vi "GUI Configuration Loop.vi"(7 "FOFB Controller IP":string, 8 "error in (no error)":errorcluster, 9 "FOFB GUI":T1, 10 "TCP Listening Timeout":i32, 11 "Configuration GUI TCP Port":u16) -> (0 "error out":errorcluster)   [LabVIEW 2011, in "User Interface VIs.lvlib"]
uses:
  User Interface VIs.lvlib
  Types Definitions/Type FOFB GUI.ctl
  Types Definitions/Type FOFB Parameters.ctl
  Types Definitions/Type Network Configuration.ctl
  Types Definitions/Type FA Configuration.ctl
  Types Definitions/Type Response Matrix Measurement Configuration.ctl
  Types Definitions/Type Correction Algorithm Configuration.ctl
  Types Definitions/Type Acquisition Network Configuration.ctl
  Types Definitions/Type Actuation Network Configuration.ctl
  Types Definitions/Type Configuration Loop Mode.ctl
  Types Definitions/Type Configuration Data (GUI to Controller).ctl
  Types Definitions/Type Monitoring Data.ctl
  Types Definitions/Type Diagnostics Data.ctl
  Types Definitions/Type CPU Loads Array.ctl
  Types Definitions/Type CPU Loads.ctl
  Types Definitions/Type Diagnostics Sample.ctl
  Types Definitions/Type Monitoring Sample.ctl
  <vilib>/Platform/TimedLoop/XDataNode/timing_clust.ctl
  <vilib>/Platform/TimedLoop/XDataNode/nitl_modes.ctl
  <vilib>/Platform/TimedLoop/XDataNode/wakeup.ctl
  Types Definitions/Type Configuration Change Acknowledge (Controller to GUI).ctl
  <vilib>/Platform/TimedLoop/XDataNode/XDataNode.xnode
  Type Definitions.lvlib
  Misc VIs.lvlib
  <vilib>/Platform/TimedLoop/XDataNode/XDNodeRunTimeDep.lvlib
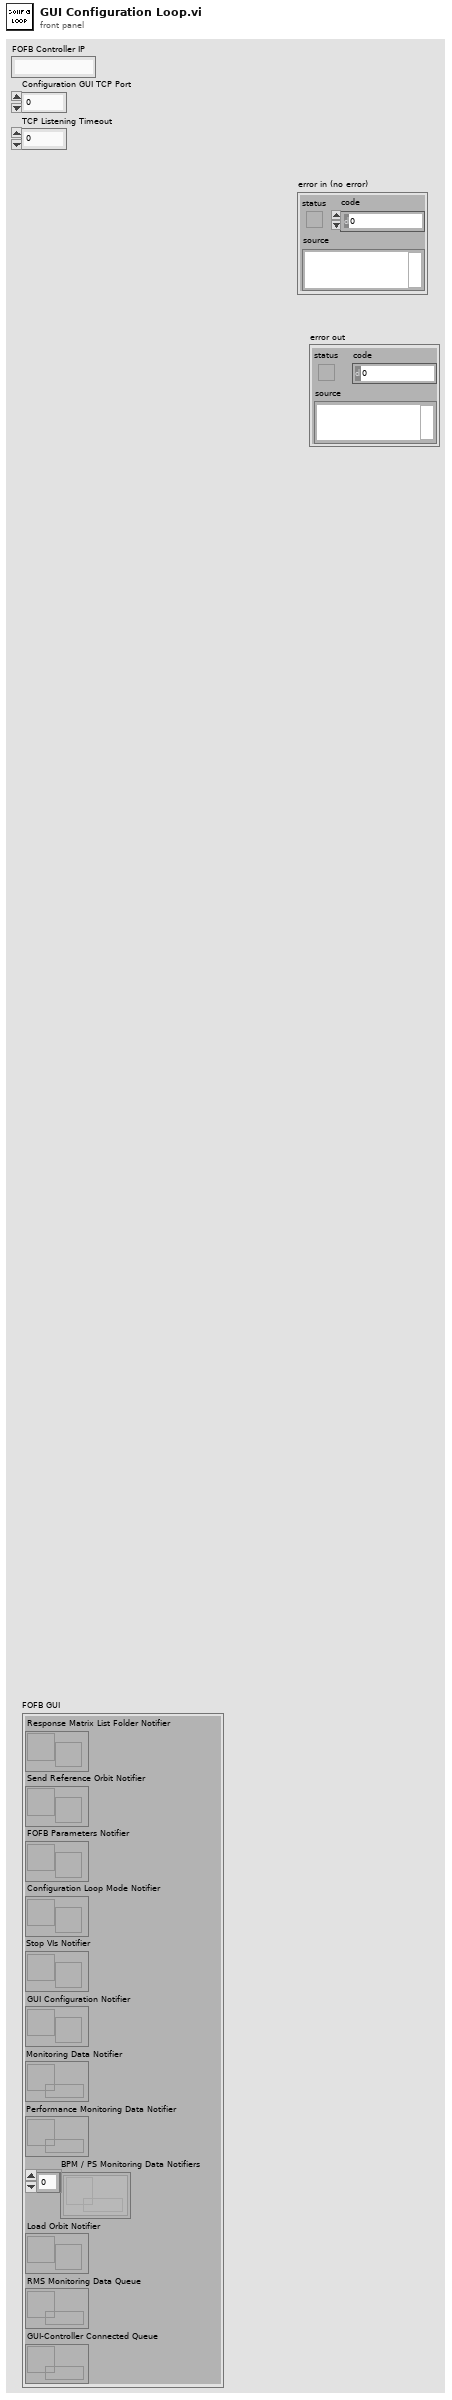
[diagram p1: front panel]
types:
  T1 = typedef "Type Definitions.lvlib/Type FOFB GUI.ctl" = cluster{"Response Matrix List Folder Notifier":refnum<notifier>, "Send Reference Orbit Notifier":refnum<notifier>, "FOFB Parameters Notifier":refnum<notifier>, "Configuration Loop Mode Notifier":refnum<notifier>, "Stop VIs Notifier":refnum<notifier>, "GUI Configuration Notifier":refnum<notifier>, "Monitoring Data Notifier":refnum<queue>, "Performance Monitoring Data Notifier":refnum<queue>, "BPM / PS Monitoring Data Notifiers":refnum<queue>[], "Load Orbit Notifier":refnum<notifier>, "RMS Monitoring Data Queue":refnum<queue>, "GUI-Controller Connected Queue":refnum<queue>}
  T2 = enum16{"Idle", "Wait Connection", "Read Data", "Process Data", "Write Data", "Close Connection"}
  T3 = typedef "XDNodeRunTimeDep.lvlib/timing_clust.ctl" = cluster{"Expected End [f-1]":u64, "Actual End [f-1]":u64, "Finished Late? [f-1]":bool, "Expected End [i-1]":u64, "Actual End [i-1]":u64, "Finished Late? [i-1]":bool, "Expected Start [i]":u64, "Actual Start [i]":u64, "Expected Start [f]":u64, "Actual Start [f]":u64, "Source Name":string, "Structure Name":string, "Period":i64, "Deadline":i64, "Offset":i64, "Start":i64, "Priority":i32, "Timeout":i32, "Mode":T4, "Wakeup Reason":T5, "Error":errorcluster, "Source Type":string, "Secondary Source Type":string, "Global End Time":u64, "Global Start Time":u64, "Frame Duration":u64, "Iteration Duration":u64, "Assigned CPU":i32, "I/O Scan Engine Mode":u32}
  T4 = typedef "XDNodeRunTimeDep.lvlib/nitl_modes.ctl" = enum32{"No Change", "Process missed periods, maintain original phase", "Discard missed periods, maintain original phase", "Process missed periods, ignore original phase", "Discard missed periods, ignore original phase"}
  T5 = typedef "XDNodeRunTimeDep.lvlib/wakeup.ctl" = enum32{"Normal", "Aborted", "Asynchronous wakeup", "Timing source error", "Timed loop error", "Timeout"}
  T6 = typedef "Type Definitions.lvlib/Type Configuration Data (GUI to Controller).ctl" = cluster{"Update Controller Soft Configuration":bool[], "Trigger RT Execution Trace":string[], "Reference Orbit":dbl[], "Request Response Matrix Folder List":bool[], "Request FOFB Parameters":bool[], "FOFB Parameters":T7[]}
  T7 = typedef "Type Definitions.lvlib/Type FOFB Parameters.ctl" = cluster{"Network":T8, "Fast Acquisition":T9, "Response Matrix Measurement":T10, "Correction Algorithm":T11, "Acquisition Network":T12, "Actuation Network":T13}
  T8 = typedef "Type Definitions.lvlib/Type Network Configuration.ctl" = cluster{"FOFB Controller IP":string, "LNLS Control Network IP":string, "LNLS Control Network Power Supplies TCP Port":u16, "LNLS Control Network FOFB Configuration TCP Port":u16, "Data Server TCP Port":u16, "Monitoring Data TCP Port":u16, "Configuration GUI TCP Port":u16, "TCP Listening Timeout":i32}
  T9 = typedef "Type Definitions.lvlib/Type FA Configuration.ctl" = cluster{"Acquisition Period":u32, "Data Buffer Size":u32, "Monitoring Period":u32}
  T10 = typedef "Type Definitions.lvlib/Type Response Matrix Measurement Configuration.ctl" = cluster{"Step Amplitude":dbl, "Time Between Steps":u32, "Step Duration":u32, "Number of Averages":u32}
  T11 = typedef "Type Definitions.lvlib/Type Correction Algorithm Configuration.ctl" = cluster{"Correction Period":u32, "Reference Orbit Path":path, "Response Matrix Path":path, "Correction Matrix Path":path, "Horizontal Correction Factor":dbl, "Vertical Correction Factor":dbl, "Beam Current FOFB Threshold":dbl, "Decouple H-V":bool, "Use Additional BPM LPF":bool, "BPM LPF Cutoff":dbl}
  T12 = typedef "Type Definitions.lvlib/Type Acquisition Network Configuration.ctl" = cluster{"Chassis Name":string, "Variables":cluster{"Variable Name":string, "Matrix Order":u32, "Location":dbl, "Plane":enum8{"H", "V"}, "On Correction":bool}[]}[]
  T13 = typedef "Type Definitions.lvlib/Type Actuation Network Configuration.ctl" = cluster{"Chassis Name":string, "Variables":cluster{"Variable Name":string, "Matrix Order":u32, "RMM Step Factor":dbl, "Plane":enum8{"H", "V"}, "On Correction":bool, "Kc":dbl, "Ti":dbl, "Td":dbl}[]}[]
  T14 = typedef "Type Definitions.lvlib/Type Configuration Change Acknowledge (Controller to GUI).ctl" = cluster{"Request Response Matrix List Folder":string[], "FOFB Parameters":T7[]}
  T15 = typedef "Type Definitions.lvlib/Type Configuration Loop Mode.ctl" = enum8{"Operation Mode", "Request FOFB Parameters", "Send New FOFB Parameters", "Send Reference Orbit", "Request Response Matrix List Folder"}
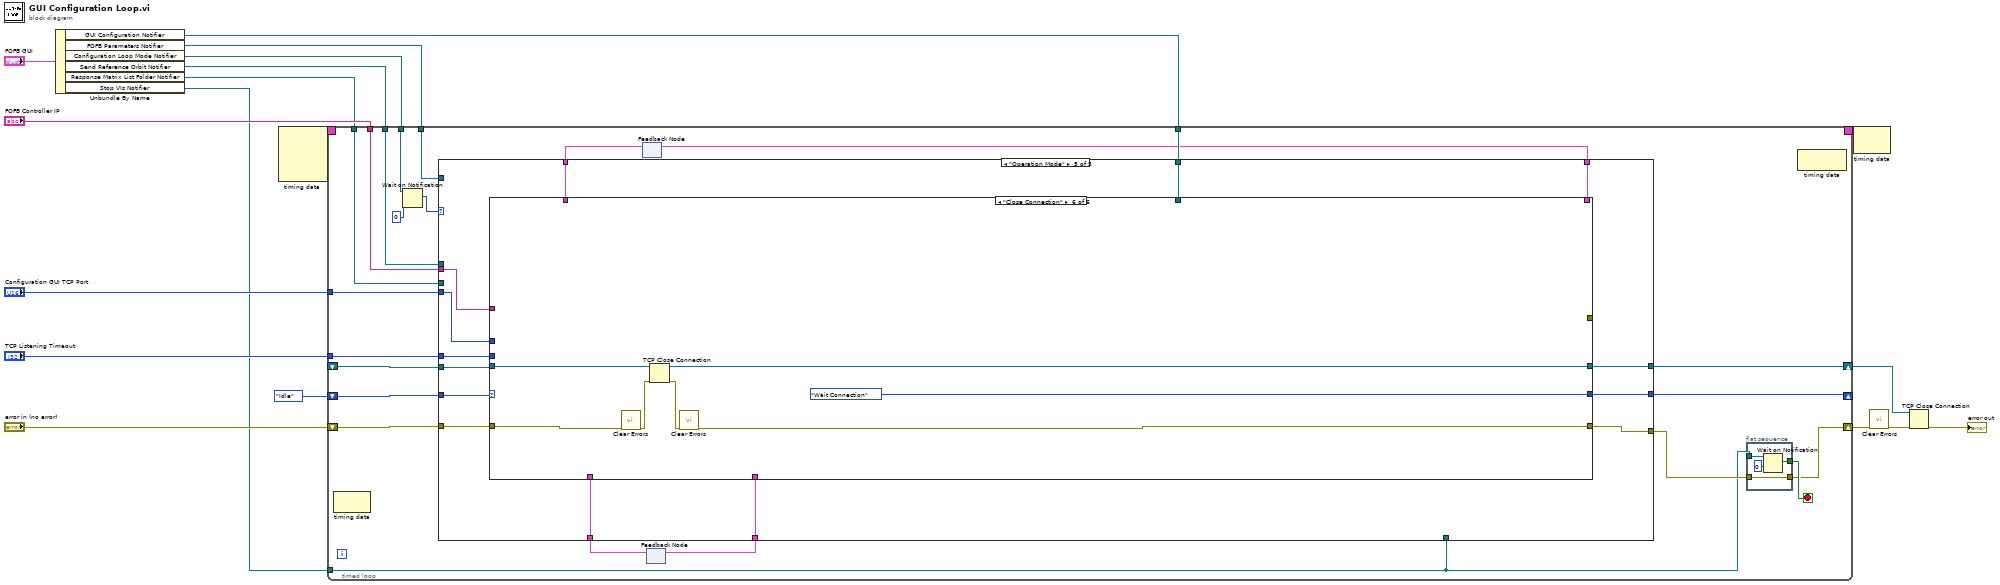
[diagram p0: block diagram]
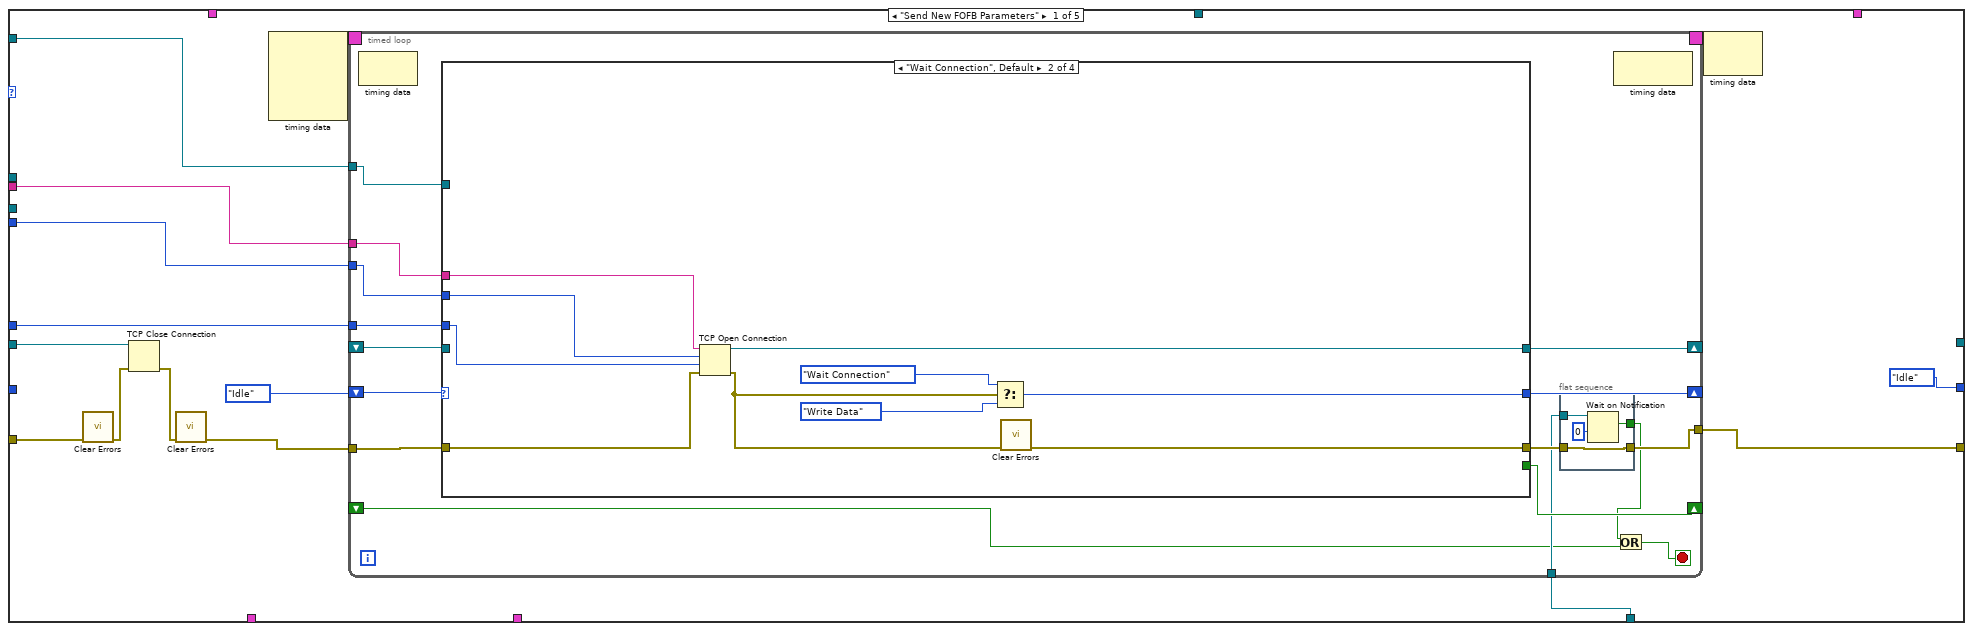
[diagram p2: hidden frame]
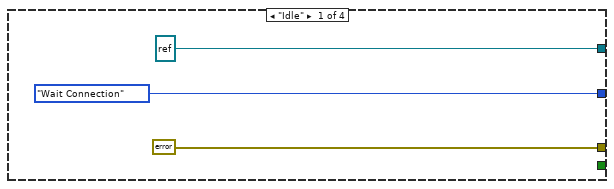
[diagram p3: hidden frame]
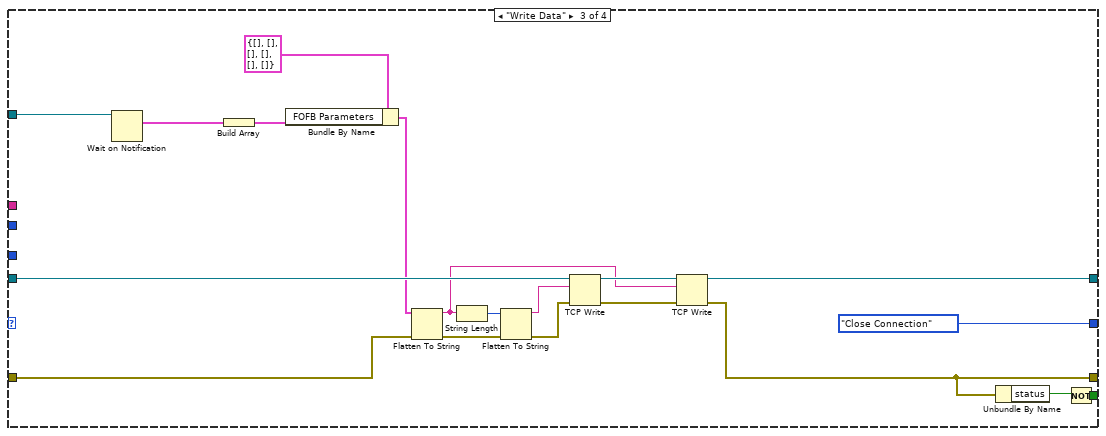
[diagram p4: hidden frame]
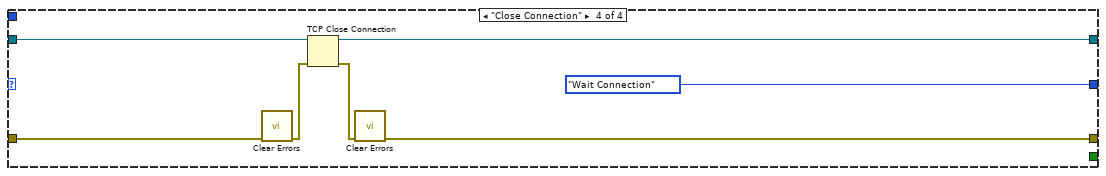
[diagram p5: hidden frame]
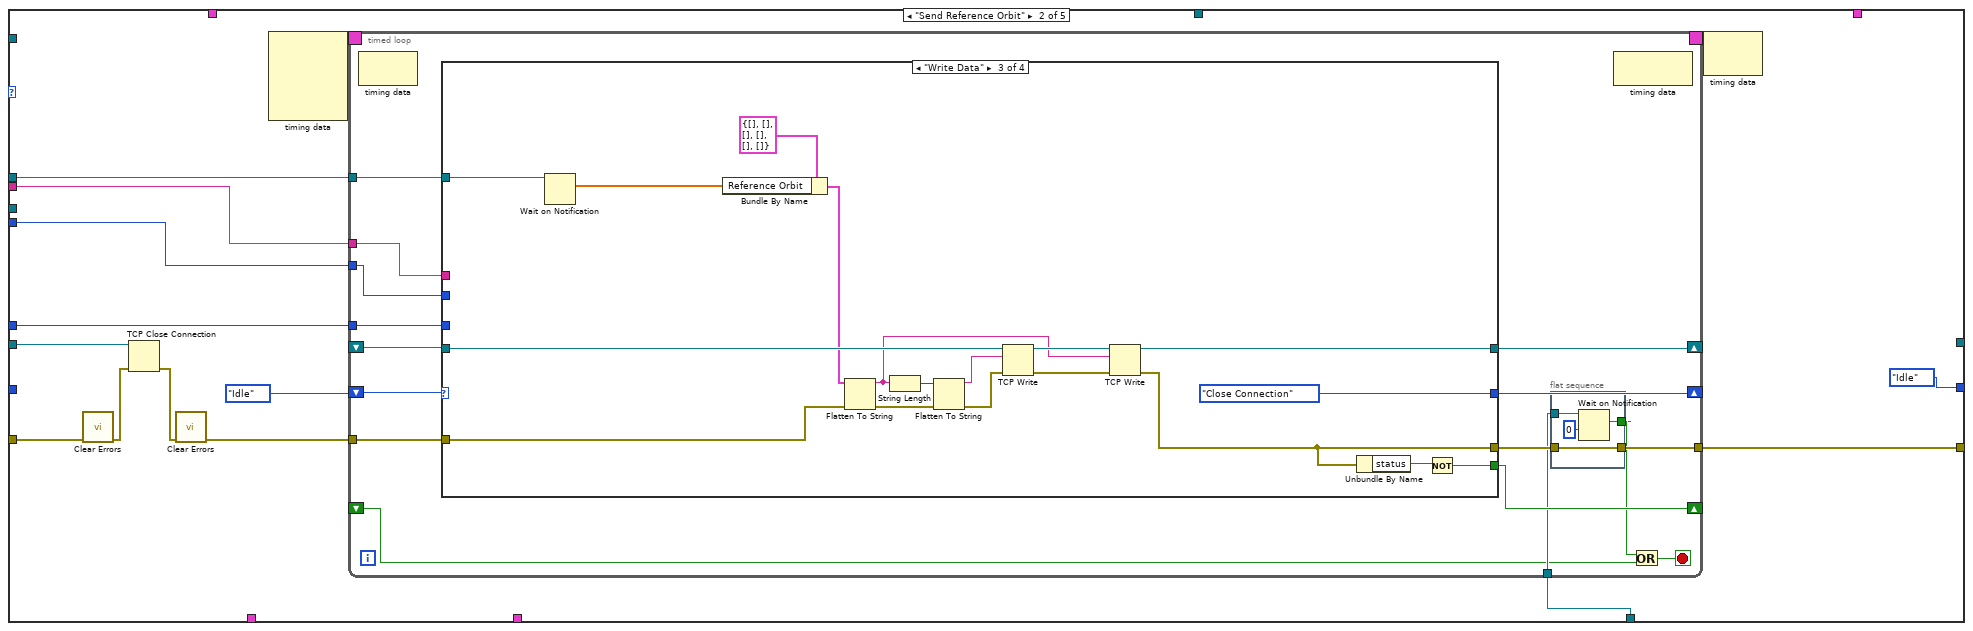
[diagram p6: hidden frame]
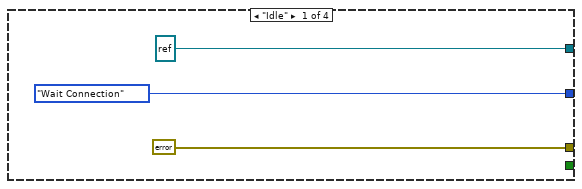
[diagram p7: hidden frame]
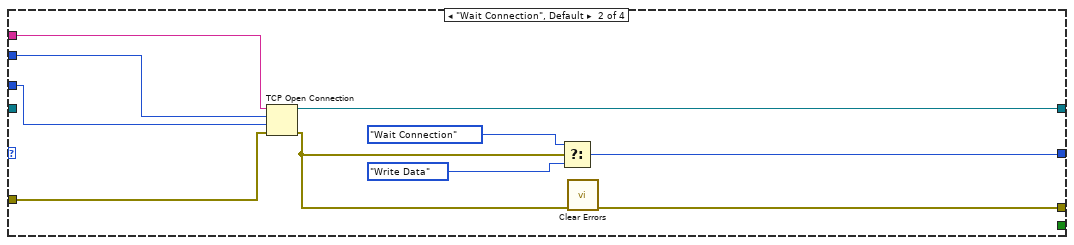
[diagram p8: hidden frame]
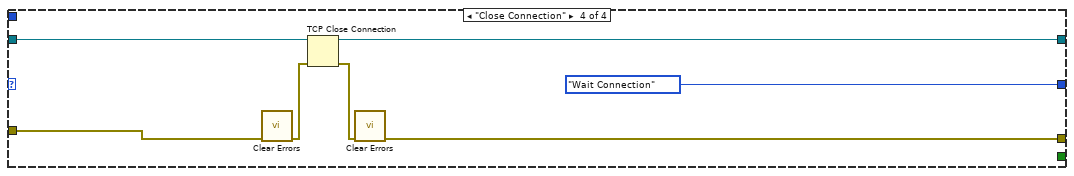
[diagram p9: hidden frame]
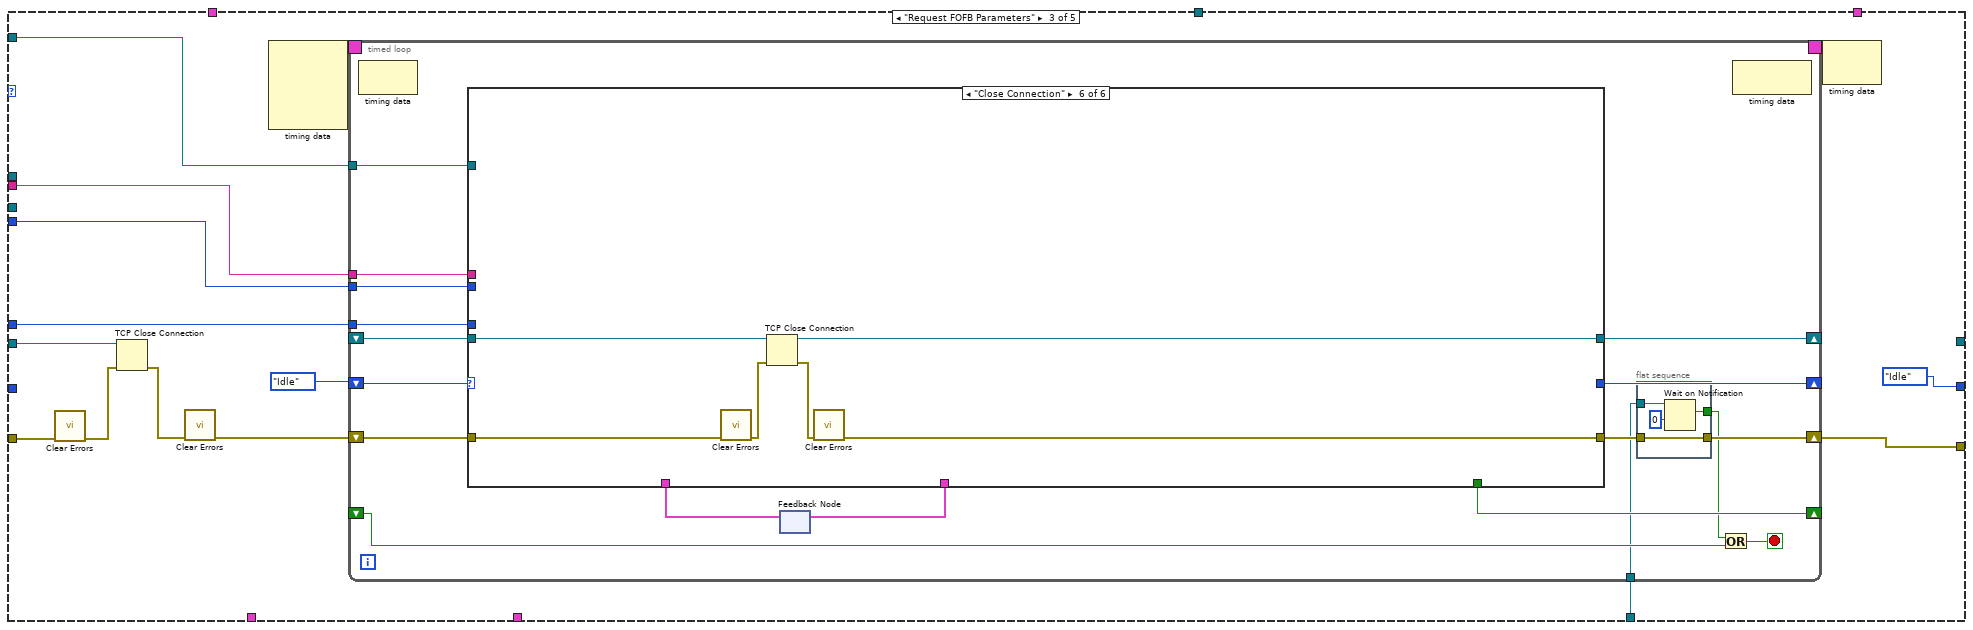
[diagram p10: hidden frame]
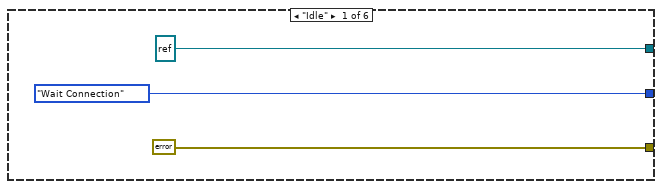
[diagram p11: hidden frame]
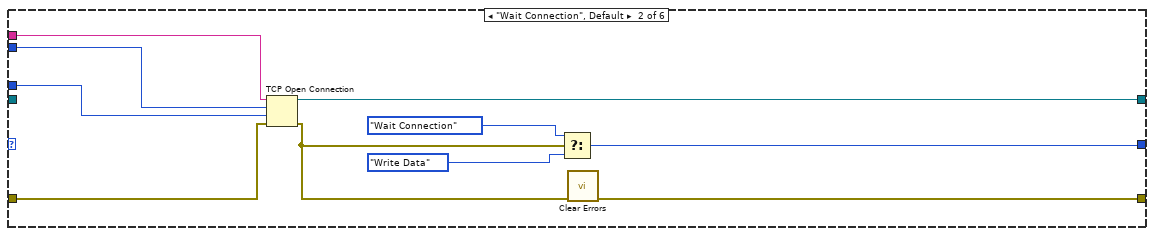
[diagram p12: hidden frame]
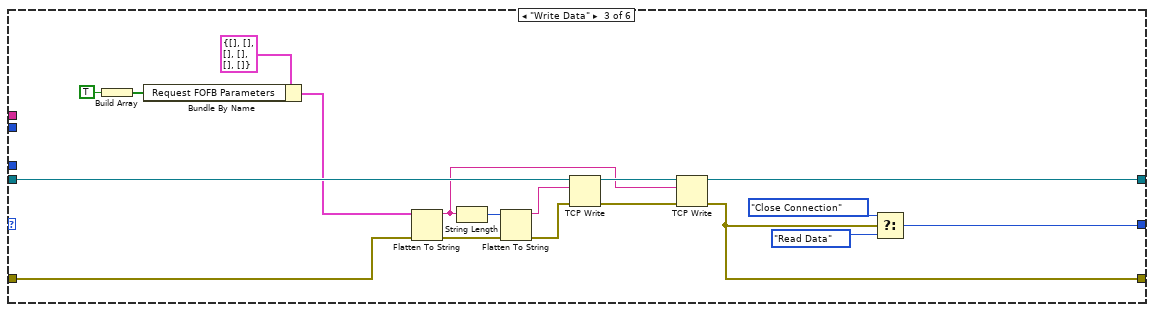
[diagram p13: hidden frame]
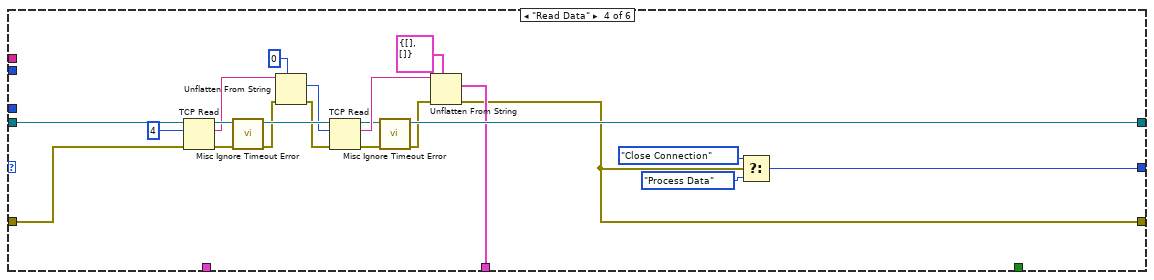
[diagram p14: hidden frame]
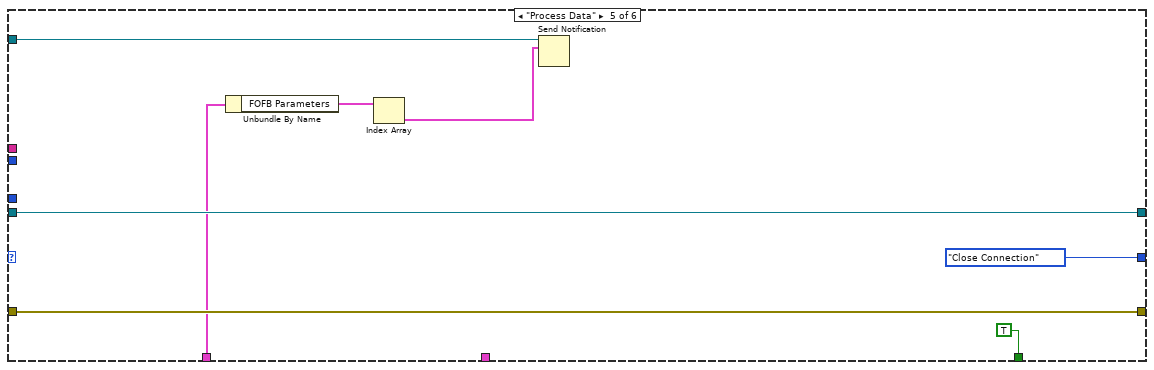
[diagram p15: hidden frame]
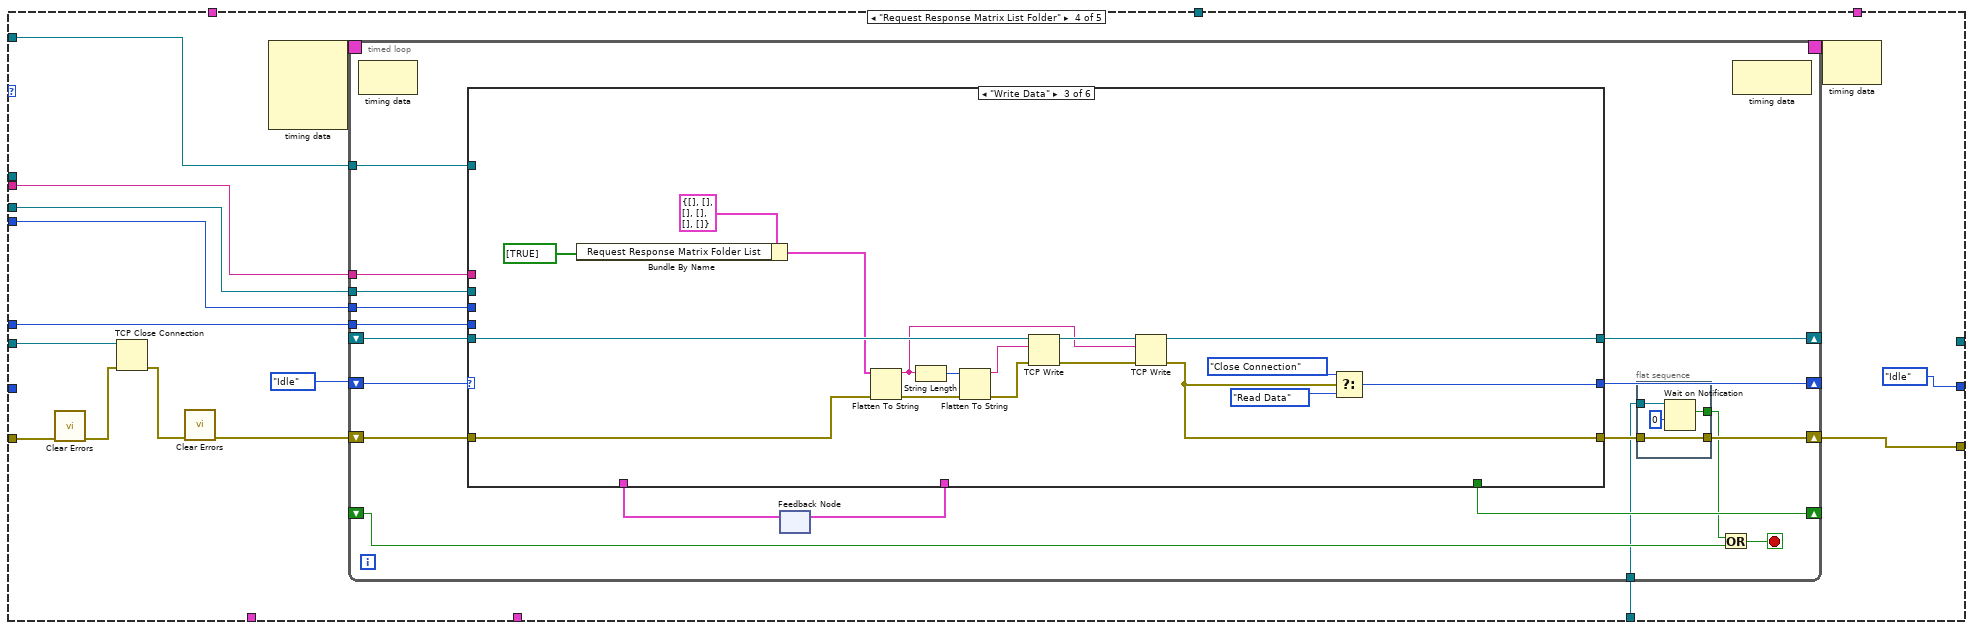
[diagram p16: hidden frame]
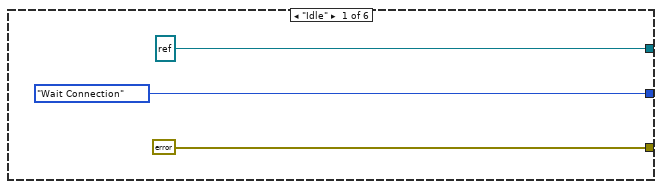
[diagram p17: hidden frame]
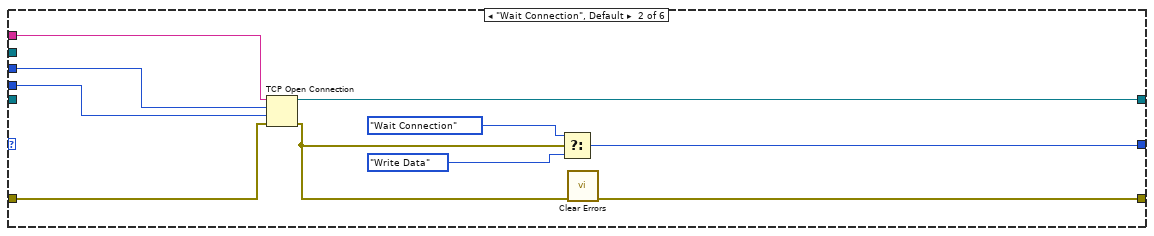
[diagram p18: hidden frame]
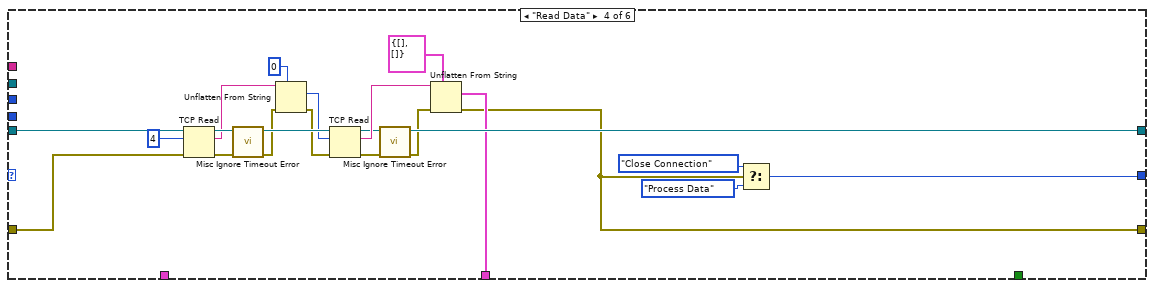
[diagram p19: hidden frame]
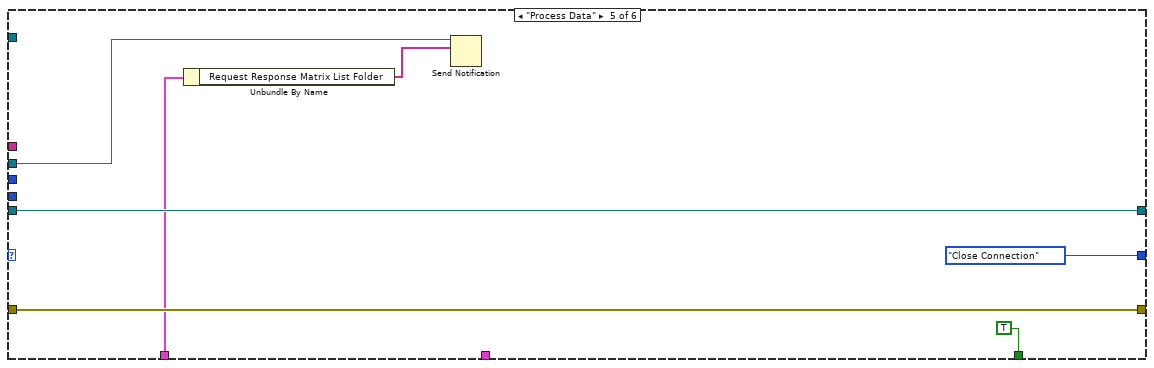
[diagram p20: hidden frame]
diagram:
  n1 = Unbundle By Name("FOFB GUI") -> ("GUI Configuration Notifier"=w9:refnum<notifier>, "FOFB Parameters Notifier"=w4:refnum<notifier>, "Configuration Loop Mode Notifier"=w12:refnum<notifier>, "Send Reference Orbit Notifier"=w3:refnum<notifier>, "Response Matrix List Folder Notifier"=w1:refnum<notifier>, "Stop VIs Notifier"=w2:refnum<notifier>)
  n2 = node-c288() -> (w16:T3)  [unwired: 4 in]
  n3 = timed-loop {
    timing: w16 -> [_]
    timing-out: [_] -> w15
    tunnel: w4 -> [w19]
    tunnel: "FOFB Controller IP" -> [w39]
    tunnel: "Configuration GUI TCP Port" -> [w38]
    tunnel: "TCP Listening Timeout" -> [w37]
    tunnel: w12 -> [w20]
    shift-right: [w33] -> w6
    shift-left: "error in (no error)" -> [w35]
    tunnel: w2 -> [w23]
    tunnel: w9 -> [w32]
    shift-right: [w30] -> _
    shift-left: T2."Idle" ("f") -> [w31]
    shift-right: [w28] -> w5
    shift-left: _ -> [w29]
    tunnel: w3 -> [w22]
    tunnel: w1 -> [w21]
    stop <- w36 stop-if-true
    n4 = node-c288() -> ()  [unwired: 1 in, 1 out]
    n5 = Wait on Notification(notifier=w20, timeout in ms (-1)=0) -> (notification=w41:T15)  [unwired: 2 in, 3 out]
    n6 = feedback #1() -> (w25:T6)  [unwired: 1 in]
    n7 = feedback #2() -> (w27:T14)  [unwired: 1 in]
    n8 = case shown="\"Operation Mode\"" w41 {
      tunnel: w35 -> [w49 w128 w203 w310 w417]
      tunnel: w19 -> [w60 _ w215 w322 _]
      tunnel: w39 -> [w56 w135 w211 w318 w420]
      tunnel: w38 -> [w55 w134 w210 w317 w419]
      tunnel: w37 -> [w54 w133 w209 w316 w418]
      tunnel: [w53 w132 w208 w315 w426] -> w34
      tunnel: w32 -> [_ _ _ _ w425]
      tunnel: w31 -> [_ _ _ _ w424]
      tunnel: [T2."Idle" ("f") T2."Idle" ("f") T2."Idle" ("f") T2."Idle" ("f") w423] -> w30
      tunnel: w29 -> [w47 w126 w204 w311 w422]
      tunnel: [_ _ _ _ w421] -> w28
      tunnel: w27 -> [_ _ _ _ w416]
      tunnel: [_ _ _ _ w415] -> w26
      tunnel: w25 -> [_ _ _ _ w414]
      tunnel: [_ _ _ _ w413] -> w24
      tunnel: w23 -> [w46 w124 w201 w308 _]
      tunnel: w22 -> [_ w125 _ _ _]
      tunnel: w21 -> [_ _ _ w307 _]
      frame "Send New FOFB Parameters" {
        n9 = call <vilib>:"Clear Errors.vi"("error in (no error)"=w49) -> ("error out"=w50:errorcluster)  [unwired: 6 in]
        n10 = TCP Close Connection(connection ID=w47, error in (no error)=w50) -> (error out=w51:errorcluster)  [unwired: 1 in, 1 out]
        n11 = call <vilib>:"Clear Errors.vi"("error in (no error)"=w51) -> ("error out"=w48:errorcluster)  [unwired: 6 in]
        n12 = node-c288() -> (w59:T3)  [unwired: 4 in]
        n13 = timed-loop {
          timing: w59 -> [_]
          timing-out: [_] -> w58
          tunnel: w48 -> [w76]
          tunnel: [w65] -> w53
          tunnel: w60 -> [w75]
          shift-right: [w71] -> _
          shift-left: T2."Idle" ("f") -> [w74]
          shift-right: [w72] -> _
          shift-left: _ -> [w73]
          tunnel: w56 -> [w70]
          tunnel: w55 -> [w69]
          tunnel: w54 -> [w68]
          shift-right: [w67] -> _
          shift-left: _ -> [w62]
          tunnel: w46 -> [w64]
          stop <- w61 stop-if-true
          n14 = node-c288() -> ()  [unwired: 1 in, 1 out]
          n15 = case shown="\"Wait Connection\", Default" w74 {
            tunnel: [refnum<k5> refnum ("connection ID") w89 w112 w119] -> w72
            tunnel: [T2."Wait Connection" ("f") w93 T2."Close Connection" ("f") T2."Wait Connection" ("f")] -> w71
            tunnel: [errorcluster {"status"=FALSE, "code"=0, "source"=""} ("error out") w92 w99 w118] -> w66
            tunnel: w76 -> [_ w87 w110 w113]
            tunnel: w73 -> [_ _ w111 w114]
            tunnel: w75 -> [_ _ w98 _]
            tunnel: w70 -> [_ w86 _ _]
            tunnel: w69 -> [_ w85 _ _]
            tunnel: w68 -> [_ w84 _ _]
            tunnel: [_ _ w100 _] -> w67
            frame "Idle" {
            }
            frame "Wait Connection", Default {
              n16 = TCP Open Connection(address=w86, remote port or service name=w85, timeout ms (60000)=w84, error in (no error)=w87) -> (connection ID=w89:refnum<k5>, error out=w88:errorcluster)  [unwired: 1 in]
              n17 = Select(t=T2."Wait Connection" ("f"), s=w88, f=T2."Write Data") -> (s? t:f=w93:T2)
              n18 = call <vilib>:"Clear Errors.vi"("error in (no error)"=w88) -> ("error out"=w92:errorcluster)  [unwired: 6 out]
            }
            frame "Write Data" {
              n19 = Wait on Notification(notifier=w98) -> (notification=w102:T7)  [unwired: 3 in, 3 out]
              n20 = Build Array(w102) -> (w94:T7[])
              n21 = Bundle By Name(cluster=T6 {"Update Controller Soft Configuration"=[], "Trigger RT Execution Trace"=[], "Reference Orbit"=[], "Request Response Matrix Folder List"=[], "Request FOFB Parameters"=[], "FOFB Parameters"=[]} ("Configuration Data (GUI to Controller)"), "FOFB Parameters"=w94) -> (w96:T6)
              n22 = Flatten To String(anything=w96, error in (no error)=w110) -> (data string=w105:string, error out=w104:errorcluster)  [unwired: 2 in, 1 out]
              n23 = String Length(string=w105) -> (length=w107:i32)
              n24 = Flatten To String(anything=w107, error in (no error)=w104) -> (data string=w106:string, error out=w103:errorcluster)  [unwired: 2 in, 1 out]
              n25 = TCP Write(connection ID=w111, data in=w106, error in (no error)=w103) -> (connection ID out=w109:refnum<k5>, error out=w108:errorcluster)  [unwired: 2 out]
              n26 = TCP Write(connection ID=w109, data in=w105, error in (no error)=w108) -> (connection ID out=w112:refnum<k5>, error out=w99:errorcluster)  [unwired: 2 out]
              n27 = Unbundle By Name(w99) -> ("status"=w101:bool)
              n28 = Not(x=w101) -> (.not. x?=w100:bool)
            }
            frame "Close Connection" {
              n29 = call <vilib>:"Clear Errors.vi"("error in (no error)"=w113) -> ("error out"=w117:errorcluster)  [unwired: 6 in]
              n30 = TCP Close Connection(connection ID=w114, error in (no error)=w117) -> (connection ID out=w119:refnum<k5>, error out=w116:errorcluster)  [unwired: 1 in]
              n31 = call <vilib>:"Clear Errors.vi"("error in (no error)"=w116) -> ("error out"=w118:errorcluster)  [unwired: 6 in]
            }
          }
          n32 = flat-sequence {
            tunnel: [w80] -> w63
            tunnel: w66 -> [w78]
            tunnel: [w78] -> w65
            tunnel: w64 -> [w77]
            frame #0 {
              n33 = Wait on Notification(notifier=w77, timeout in ms (-1)=0) -> (notification=w80:bool)  [unwired: 2 in, 3 out]
            }
          }
          n34 = node-c288() -> ()  [unwired: 1 in, 1 out]
          n35 = Or(x=w63, y=w62) -> (x .or. y?=w61:bool)
        }
        n36 = node-c288(w58) -> ()  [unwired: 1 out]
      }
      frame "Send Reference Orbit" {
        n37 = call <vilib>:"Clear Errors.vi"("error in (no error)"=w128) -> ("error out"=w129:errorcluster)  [unwired: 6 in]
        n38 = TCP Close Connection(connection ID=w126, error in (no error)=w129) -> (error out=w130:errorcluster)  [unwired: 1 in, 1 out]
        n39 = call <vilib>:"Clear Errors.vi"("error in (no error)"=w130) -> ("error out"=w127:errorcluster)  [unwired: 6 in]
        n40 = node-c288() -> (w138:T3)  [unwired: 4 in]
        n41 = timed-loop {
          timing: w138 -> [_]
          timing-out: [_] -> w137
          tunnel: w127 -> [w154]
          tunnel: [w143] -> w132
          shift-right: [w150] -> _
          shift-left: T2."Idle" ("f") -> [w153]
          shift-right: [w151] -> _
          shift-left: _ -> [w152]
          tunnel: w135 -> [w149]
          tunnel: w134 -> [w148]
          tunnel: w133 -> [w147]
          shift-right: [w146] -> _
          shift-left: _ -> [w140]
          tunnel: w125 -> [w145]
          tunnel: w124 -> [w142]
          stop <- w139 stop-if-true
          n42 = node-c288() -> ()  [unwired: 1 in, 1 out]
          n43 = case shown="\"Write Data\"" w153 {
            tunnel: [refnum<k5> refnum ("connection ID") w167 w189 w196] -> w151
            tunnel: [T2."Wait Connection" ("f") w171 T2."Close Connection" ("f") T2."Wait Connection" ("f")] -> w150
            tunnel: [errorcluster {"status"=FALSE, "code"=0, "source"=""} ("error out") w170 w177 w195] -> w144
            tunnel: w154 -> [_ w165 w187 w190]
            tunnel: w152 -> [_ _ w188 w191]
            tunnel: w149 -> [_ w164 _ _]
            tunnel: w148 -> [_ w163 _ _]
            tunnel: w147 -> [_ w162 _ _]
            tunnel: [_ _ w178 _] -> w146
            tunnel: w145 -> [_ _ w173 _]
            frame "Idle" {
            }
            frame "Wait Connection", Default {
              n44 = TCP Open Connection(address=w164, remote port or service name=w163, timeout ms (60000)=w162, error in (no error)=w165) -> (connection ID=w167:refnum<k5>, error out=w166:errorcluster)  [unwired: 1 in]
              n45 = Select(t=T2."Wait Connection" ("f"), s=w166, f=T2."Write Data") -> (s? t:f=w171:T2)
              n46 = call <vilib>:"Clear Errors.vi"("error in (no error)"=w166) -> ("error out"=w170:errorcluster)  [unwired: 6 out]
            }
            frame "Write Data" {
              n47 = Wait on Notification(notifier=w173) -> (notification=w172:dbl[])  [unwired: 3 in, 3 out]
              n48 = Bundle By Name(cluster=T6 {"Update Controller Soft Configuration"=[], "Trigger RT Execution Trace"=[], "Reference Orbit"=[], "Request Response Matrix Folder List"=[], "Request FOFB Parameters"=[], "FOFB Parameters"=[]} ("Configuration Data (GUI to Controller)"), "Reference Orbit"=w172) -> (w174:T6)
              n49 = Flatten To String(anything=w174, error in (no error)=w187) -> (data string=w182:string, error out=w181:errorcluster)  [unwired: 2 in, 1 out]
              n50 = String Length(string=w182) -> (length=w184:i32)
              n51 = Flatten To String(anything=w184, error in (no error)=w181) -> (data string=w183:string, error out=w180:errorcluster)  [unwired: 2 in, 1 out]
              n52 = TCP Write(connection ID=w188, data in=w183, error in (no error)=w180) -> (connection ID out=w186:refnum<k5>, error out=w185:errorcluster)  [unwired: 2 out]
              n53 = TCP Write(connection ID=w186, data in=w182, error in (no error)=w185) -> (connection ID out=w189:refnum<k5>, error out=w177:errorcluster)  [unwired: 2 out]
              n54 = Unbundle By Name(w177) -> ("status"=w179:bool)
              n55 = Not(x=w179) -> (.not. x?=w178:bool)
            }
            frame "Close Connection" {
              n56 = call <vilib>:"Clear Errors.vi"("error in (no error)"=w190) -> ("error out"=w194:errorcluster)  [unwired: 6 in]
              n57 = TCP Close Connection(connection ID=w191, error in (no error)=w194) -> (connection ID out=w196:refnum<k5>, error out=w193:errorcluster)  [unwired: 1 in]
              n58 = call <vilib>:"Clear Errors.vi"("error in (no error)"=w193) -> ("error out"=w195:errorcluster)  [unwired: 6 in]
            }
          }
          n59 = flat-sequence {
            tunnel: [w158] -> w143
            tunnel: w144 -> [w158]
            tunnel: w142 -> [w157]
            tunnel: [w155] -> _
            tunnel: [w155] -> w141
            frame #0 {
              n60 = Wait on Notification(notifier=w157, timeout in ms (-1)=0) -> (notification=w155:bool)  [unwired: 2 in, 3 out]
            }
          }
          n61 = node-c288() -> ()  [unwired: 1 in, 1 out]
          n62 = Or(x=w141, y=w140) -> (x .or. y?=w139:bool)
        }
        n63 = node-c288(w137) -> ()  [unwired: 1 out]
      }
      frame "Request FOFB Parameters" {
        n64 = call <vilib>:"Clear Errors.vi"("error in (no error)"=w203) -> ("error out"=w206:errorcluster)  [unwired: 6 in]
        n65 = TCP Close Connection(connection ID=w204, error in (no error)=w206) -> (error out=w205:errorcluster)  [unwired: 1 in, 1 out]
        n66 = call <vilib>:"Clear Errors.vi"("error in (no error)"=w205) -> ("error out"=w202:errorcluster)  [unwired: 6 in]
        n67 = node-c288() -> (w214:T3)  [unwired: 4 in]
        n68 = timed-loop {
          timing: w214 -> [_]
          timing-out: [_] -> w213
          tunnel: w215 -> [w231]
          shift-right: [w230] -> _
          shift-left: T2."Idle" ("f") -> [w229]
          shift-right: [w228] -> _
          shift-left: _ -> [w227]
          tunnel: w211 -> [w226]
          tunnel: w210 -> [w225]
          tunnel: w209 -> [w224]
          shift-right: [w223] -> _
          shift-left: _ -> [w217]
          shift-right: [w220] -> w208
          shift-left: w202 -> [w222]
          tunnel: w201 -> [w216]
          stop <- w218 stop-if-true
          n69 = node-c288() -> ()  [unwired: 1 in, 1 out]
          n70 = feedback #3() -> (w232:T14)  [unwired: 1 in]
          n71 = case shown="\"Close Connection\"" w229 {
            tunnel: [refnum<k5> refnum ("connection ID") w246 w268 w281 w295 w302] -> w228
            tunnel: [T2."Wait Connection" ("f") w250 w267 w277 T2."Close Connection" ("f") _] -> w230
            tunnel: [errorcluster {"status"=FALSE, "code"=0, "source"=""} ("error out") w249 w266 w269 w296 w301] -> w221
            tunnel: w222 -> [_ w244 w264 w280 w296 w297]
            tunnel: w227 -> [_ _ w265 w282 w295 w298]
            tunnel: [_ _ _ w273 _ _] -> w233
            tunnel: w232 -> [_ _ _ _ w293 _]
            tunnel: w231 -> [_ _ _ _ w294 _]
            tunnel: w226 -> [_ w243 _ _ _ _]
            tunnel: w225 -> [_ w242 _ _ _ _]
            tunnel: w224 -> [_ w241 _ _ _ _]
            tunnel: [_ _ _ _ TRUE _] -> w223
            frame "Idle" {
            }
            frame "Wait Connection", Default {
              n72 = TCP Open Connection(address=w243, remote port or service name=w242, timeout ms (60000)=w241, error in (no error)=w244) -> (connection ID=w246:refnum<k5>, error out=w245:errorcluster)  [unwired: 1 in]
              n73 = Select(t=T2."Wait Connection" ("f"), s=w245, f=T2."Write Data") -> (s? t:f=w250:T2)
              n74 = call <vilib>:"Clear Errors.vi"("error in (no error)"=w245) -> ("error out"=w249:errorcluster)  [unwired: 6 out]
            }
            frame "Write Data" {
              n75 = Build Array(TRUE) -> (w253:bool[])
              n76 = Bundle By Name(cluster=T6 {"Update Controller Soft Configuration"=[], "Trigger RT Execution Trace"=[], "Reference Orbit"=[], "Request Response Matrix Folder List"=[], "Request FOFB Parameters"=[], "FOFB Parameters"=[]} ("Configuration Data (GUI to Controller)"), "Request FOFB Parameters"=w253) -> (w254:T6)
              n77 = Flatten To String(anything=w254, error in (no error)=w264) -> (data string=w259:string, error out=w256:errorcluster)  [unwired: 2 in, 1 out]
              n78 = String Length(string=w259) -> (length=w261:i32)
              n79 = Flatten To String(anything=w261, error in (no error)=w256) -> (data string=w260:string, error out=w255:errorcluster)  [unwired: 2 in, 1 out]
              n80 = TCP Write(connection ID=w265, data in=w260, error in (no error)=w255) -> (connection ID out=w263:refnum<k5>, error out=w262:errorcluster)  [unwired: 2 out]
              n81 = TCP Write(connection ID=w263, data in=w259, error in (no error)=w262) -> (connection ID out=w268:refnum<k5>, error out=w266:errorcluster)  [unwired: 2 out]
              n82 = Select(t=T2."Close Connection" ("f"), s=w266, f=T2."Read Data") -> (s? t:f=w267:T2)
            }
            frame "Read Data" {
              n83 = TCP Read(connection ID=w282, bytes to read=4, error in (no error)=w280) -> (connection ID out=w288:refnum<k5>, data out=w286:string, error out=w275:errorcluster)  [unwired: 2 in]
              n84 = call "Misc Ignore Timeout Error.vi"("error in (no error)"=w275) -> ("error out"=w272:errorcluster)  [unwired: 10 in]
              n85 = Unflatten From String(type=0 ("bytes to read"), binary string=w286, error in (no error)=w272) -> (value=w284:i32, error out=w271:errorcluster)  [unwired: 2 in, 1 out]
              n86 = TCP Read(connection ID=w288, bytes to read=w284, error in (no error)=w271) -> (connection ID out=w281:refnum<k5>, data out=w283:string, error out=w274:errorcluster)  [unwired: 2 in]
              n87 = call "Misc Ignore Timeout Error.vi"("error in (no error)"=w274) -> ("error out"=w270:errorcluster)  [unwired: 10 in]
              n88 = Unflatten From String(type=T14 {"Request Response Matrix List Folder"=[], "FOFB Parameters"=[]} ("Configuration Change Acknowledge (Controller to GUI)"), binary string=w283, error in (no error)=w270) -> (value=w273:T14, error out=w269:errorcluster)  [unwired: 2 in, 1 out]
              n89 = Select(t=T2."Close Connection" ("f"), s=w269, f=T2."Process Data") -> (s? t:f=w277:T2)
            }
            frame "Process Data" {
              n90 = Unbundle By Name(w293) -> ("FOFB Parameters"=w292:T7[])
              n91 = Index Array(array=w292) -> (element=w291:T7)  [unwired: 1 in]
              n92 = Send Notification(notification=w291, notifier=w294) -> ()  [unwired: 1 in, 2 out]
            }
            frame "Close Connection" {
              n93 = call <vilib>:"Clear Errors.vi"("error in (no error)"=w297) -> ("error out"=w300:errorcluster)  [unwired: 6 in]
              n94 = TCP Close Connection(connection ID=w298, error in (no error)=w300) -> (connection ID out=w302:refnum<k5>, error out=w299:errorcluster)  [unwired: 1 in]
              n95 = call <vilib>:"Clear Errors.vi"("error in (no error)"=w299) -> ("error out"=w301:errorcluster)  [unwired: 6 in]
            }
          }
          n96 = feedback-in #3(w233) -> ()
          n97 = flat-sequence {
            tunnel: [w237] -> w220
            tunnel: w221 -> [w237]
            tunnel: w216 -> [w236]
            tunnel: [w235] -> w219
            frame #0 {
              n98 = Wait on Notification(notifier=w236, timeout in ms (-1)=0) -> (notification=w235:bool)  [unwired: 2 in, 3 out]
            }
          }
          n99 = Or(x=w219, y=w217) -> (x .or. y?=w218:bool)
          n100 = node-c288() -> ()  [unwired: 1 in, 1 out]
        }
        n101 = node-c288(w213) -> ()  [unwired: 1 out]
      }
      frame "Request Response Matrix List Folder" {
        n102 = call <vilib>:"Clear Errors.vi"("error in (no error)"=w310) -> ("error out"=w313:errorcluster)  [unwired: 6 in]
        n103 = TCP Close Connection(connection ID=w311, error in (no error)=w313) -> (error out=w312:errorcluster)  [unwired: 1 in, 1 out]
        n104 = call <vilib>:"Clear Errors.vi"("error in (no error)"=w312) -> ("error out"=w309:errorcluster)  [unwired: 6 in]
        n105 = node-c288() -> (w321:T3)  [unwired: 4 in]
        n106 = timed-loop {
          timing: w321 -> [_]
          timing-out: [_] -> w320
          tunnel: w322 -> [w339]
          shift-right: [w338] -> _
          shift-left: T2."Idle" ("f") -> [w337]
          shift-right: [w336] -> _
          shift-left: _ -> [w335]
          tunnel: w318 -> [w334]
          tunnel: w317 -> [w333]
          tunnel: w316 -> [w332]
          shift-right: [w331] -> _
          shift-left: _ -> [w325]
          shift-right: [w328] -> w315
          shift-left: w309 -> [w330]
          tunnel: w308 -> [w324]
          tunnel: w307 -> [w323]
          stop <- w326 stop-if-true
          n107 = node-c288() -> ()  [unwired: 1 in, 1 out]
          n108 = feedback #4() -> (w340:T14)  [unwired: 1 in]
          n109 = case shown="\"Write Data\"" w337 {
            tunnel: [refnum<k5> refnum ("connection ID") w354 w375 w388 w401 w408] -> w336
            tunnel: [T2."Wait Connection" ("f") w358 w374 w384 T2."Close Connection" ("f") _] -> w338
            tunnel: [errorcluster {"status"=FALSE, "code"=0, "source"=""} ("error out") w357 w373 w376 w402 w407] -> w329
            tunnel: w330 -> [_ w352 w371 w387 w402 w403]
            tunnel: w335 -> [_ _ w372 w389 w401 w404]
            tunnel: [_ _ _ w380 _ _] -> w341
            tunnel: w340 -> [_ _ _ _ w397 _]
            tunnel: w339 -> [_ _ _ _ _ _]
            tunnel: w334 -> [_ w351 _ _ _ _]
            tunnel: w333 -> [_ w350 _ _ _ _]
            tunnel: w332 -> [_ w349 _ _ _ _]
            tunnel: [_ _ _ _ TRUE _] -> w331
            tunnel: w323 -> [_ _ _ _ w398 _]
            frame "Idle" {
            }
            frame "Wait Connection", Default {
              n110 = TCP Open Connection(address=w351, remote port or service name=w350, timeout ms (60000)=w349, error in (no error)=w352) -> (connection ID=w354:refnum<k5>, error out=w353:errorcluster)  [unwired: 1 in]
              n111 = Select(t=T2."Wait Connection" ("f"), s=w353, f=T2."Write Data") -> (s? t:f=w358:T2)
              n112 = call <vilib>:"Clear Errors.vi"("error in (no error)"=w353) -> ("error out"=w357:errorcluster)  [unwired: 6 out]
            }
            frame "Write Data" {
              n113 = Bundle By Name(cluster=T6 {"Update Controller Soft Configuration"=[], "Trigger RT Execution Trace"=[], "Reference Orbit"=[], "Request Response Matrix Folder List"=[], "Request FOFB Parameters"=[], "FOFB Parameters"=[]} ("Configuration Data (GUI to Controller)"), "Request Response Matrix Folder List"=bool[] [TRUE] ("Request Folder List")) -> (w361:T6)
              n114 = Flatten To String(anything=w361, error in (no error)=w371) -> (data string=w366:string, error out=w363:errorcluster)  [unwired: 2 in, 1 out]
              n115 = String Length(string=w366) -> (length=w368:i32)
              n116 = Flatten To String(anything=w368, error in (no error)=w363) -> (data string=w367:string, error out=w362:errorcluster)  [unwired: 2 in, 1 out]
              n117 = TCP Write(connection ID=w372, data in=w367, error in (no error)=w362) -> (connection ID out=w370:refnum<k5>, error out=w369:errorcluster)  [unwired: 2 out]
              n118 = TCP Write(connection ID=w370, data in=w366, error in (no error)=w369) -> (connection ID out=w375:refnum<k5>, error out=w373:errorcluster)  [unwired: 2 out]
              n119 = Select(t=T2."Close Connection" ("f"), s=w373, f=T2."Read Data") -> (s? t:f=w374:T2)
            }
            frame "Read Data" {
              n120 = TCP Read(connection ID=w389, bytes to read=4, error in (no error)=w387) -> (connection ID out=w395:refnum<k5>, data out=w393:string, error out=w382:errorcluster)  [unwired: 2 in]
              n121 = call "Misc Ignore Timeout Error.vi"("error in (no error)"=w382) -> ("error out"=w379:errorcluster)  [unwired: 10 in]
              n122 = Unflatten From String(type=0 ("bytes to read"), binary string=w393, error in (no error)=w379) -> (value=w391:i32, error out=w378:errorcluster)  [unwired: 2 in, 1 out]
              n123 = TCP Read(connection ID=w395, bytes to read=w391, error in (no error)=w378) -> (connection ID out=w388:refnum<k5>, data out=w390:string, error out=w381:errorcluster)  [unwired: 2 in]
              n124 = call "Misc Ignore Timeout Error.vi"("error in (no error)"=w381) -> ("error out"=w377:errorcluster)  [unwired: 10 in]
              n125 = Unflatten From String(type=T14 {"Request Response Matrix List Folder"=[], "FOFB Parameters"=[]} ("Configuration Change Acknowledge (Controller to GUI)"), binary string=w390, error in (no error)=w377) -> (value=w380:T14, error out=w376:errorcluster)  [unwired: 2 in, 1 out]
              n126 = Select(t=T2."Close Connection" ("f"), s=w376, f=T2."Process Data") -> (s? t:f=w384:T2)
            }
            frame "Process Data" {
              n127 = Unbundle By Name(w397) -> ("Request Response Matrix List Folder"=w396:string[])
              n128 = Send Notification(notification=w396, notifier=w398) -> ()  [unwired: 1 in, 2 out]
            }
            frame "Close Connection" {
              n129 = call <vilib>:"Clear Errors.vi"("error in (no error)"=w403) -> ("error out"=w406:errorcluster)  [unwired: 6 in]
              n130 = TCP Close Connection(connection ID=w404, error in (no error)=w406) -> (connection ID out=w408:refnum<k5>, error out=w405:errorcluster)  [unwired: 1 in]
              n131 = call <vilib>:"Clear Errors.vi"("error in (no error)"=w405) -> ("error out"=w407:errorcluster)  [unwired: 6 in]
            }
          }
          n132 = feedback-in #4(w341) -> ()
          n133 = flat-sequence {
            tunnel: [w345] -> w328
            tunnel: w329 -> [w345]
            tunnel: w324 -> [w344]
            tunnel: [w343] -> w327
            frame #0 {
              n134 = Wait on Notification(notifier=w344, timeout in ms (-1)=0) -> (notification=w343:bool)  [unwired: 2 in, 3 out]
            }
          }
          n135 = Or(x=w327, y=w325) -> (x .or. y?=w326:bool)
          n136 = node-c288() -> ()  [unwired: 1 in, 1 out]
        }
        n137 = node-c288(w320) -> ()  [unwired: 1 out]
      }
      frame "Operation Mode" {
        n138 = case shown="\"Close Connection\"" w424 {
          tunnel: [refnum<k5> refnum ("connection ID") w435 w446 w461 w474 w488] -> w421
          tunnel: [T2."Wait Connection" ("f") w439 T2."Write Data" ("f") w460 w470 T2."Wait Connection" ("f")] -> w423
          tunnel: [errorcluster {"status"=FALSE, "code"=0, "source"=""} ("error out") w438 w440 w459 w462 w487] -> w426
          tunnel: w417 -> [_ w433 w440 w448 w473 w482]
          tunnel: w422 -> [_ _ w446 w457 w475 w483]
          tunnel: [_ _ _ _ w466 _] -> w415
          tunnel: w416 -> [_ _ _ _ _ _]
          tunnel: [_ _ w442 _ _ _] -> w413
          tunnel: w414 -> [_ _ _ w450 _ _]
          tunnel: w420 -> [_ w432 _ _ _ _]
          tunnel: w419 -> [_ w431 _ _ _ _]
          tunnel: w418 -> [_ w430 _ _ _ _]
          tunnel: w425 -> [_ _ w444 _ _ _]
          tunnel: [_ _ w441 _ _ _] -> _
          frame "Idle" {
          }
          frame "Wait Connection", Default {
            n139 = TCP Open Connection(address=w432, remote port or service name=w431, timeout ms (60000)=w430, error in (no error)=w433) -> (connection ID=w435:refnum<k5>, error out=w434:errorcluster)  [unwired: 1 in]
            n140 = Select(t=T2."Wait Connection" ("f"), s=w434, f=T2."Process Data") -> (s? t:f=w439:T2)
            n141 = call <vilib>:"Clear Errors.vi"("error in (no error)"=w434) -> ("error out"=w438:errorcluster)  [unwired: 6 out]
          }
          frame "Process Data" {
            n142 = Wait on Notification(notifier=w444, timeout in ms (-1)=200) -> (notification=w442:T6, error out=w441:errorcluster)  [unwired: 2 in, 2 out]
          }
          frame "Write Data" {
            n143 = Flatten To String(anything=w450, error in (no error)=w448) -> (data string=w453:string, error out=w449:errorcluster)  [unwired: 2 in, 1 out]
            n144 = String Length(string=w453) -> (length=w455:i32)
            n145 = Flatten To String(anything=w455, error in (no error)=w449) -> (data string=w454:string, error out=w447:errorcluster)  [unwired: 2 in, 1 out]
            n146 = TCP Write(connection ID=w457, data in=w454, error in (no error)=w447) -> (connection ID out=w458:refnum<k5>, error out=w456:errorcluster)  [unwired: 2 out]
            n147 = TCP Write(connection ID=w458, data in=w453, error in (no error)=w456) -> (connection ID out=w461:refnum<k5>, error out=w459:errorcluster)  [unwired: 2 out]
            n148 = Select(t=T2."Close Connection" ("f"), s=w459, f=T2."Read Data") -> (s? t:f=w460:T2)
          }
          frame "Read Data" {
            n149 = TCP Read(connection ID=w475, bytes to read=4, error in (no error)=w473) -> (connection ID out=w481:refnum<k5>, data out=w479:string, error out=w468:errorcluster)  [unwired: 2 in]
            n150 = call "Misc Ignore Timeout Error.vi"("error in (no error)"=w468) -> ("error out"=w465:errorcluster)  [unwired: 10 in]
            n151 = Unflatten From String(type=0 ("bytes to read"), binary string=w479, error in (no error)=w465) -> (value=w477:i32, error out=w464:errorcluster)  [unwired: 2 in, 1 out]
            n152 = TCP Read(connection ID=w481, bytes to read=w477, error in (no error)=w464) -> (connection ID out=w474:refnum<k5>, data out=w476:string, error out=w467:errorcluster)  [unwired: 2 in]
            n153 = call "Misc Ignore Timeout Error.vi"("error in (no error)"=w467) -> ("error out"=w463:errorcluster)  [unwired: 10 in]
            n154 = Unflatten From String(type=T14 {"Request Response Matrix List Folder"=[], "FOFB Parameters"=[]} ("Configuration Change Acknowledge (Controller to GUI)"), binary string=w476, error in (no error)=w463) -> (value=w466:T14, error out=w462:errorcluster)  [unwired: 2 in, 1 out]
            n155 = Select(t=T2."Close Connection" ("f"), s=w462, f=T2."Process Data") -> (s? t:f=w470:T2)
          }
          frame "Close Connection" {
            n156 = call <vilib>:"Clear Errors.vi"("error in (no error)"=w482) -> ("error out"=w486:errorcluster)  [unwired: 6 in]
            n157 = TCP Close Connection(connection ID=w483, error in (no error)=w486) -> (connection ID out=w488:refnum<k5>, error out=w485:errorcluster)  [unwired: 1 in]
            n158 = call <vilib>:"Clear Errors.vi"("error in (no error)"=w485) -> ("error out"=w487:errorcluster)  [unwired: 6 in]
          }
        }
      }
    }
    n159 = feedback-in #1(w24) -> ()
    n160 = feedback-in #2(w26) -> ()
    n161 = flat-sequence {
      tunnel: [w45] -> w33
      tunnel: w34 -> [w45]
      tunnel: w23 -> [w44]
      tunnel: [w43] -> w36
      frame #0 {
        n162 = Wait on Notification(notifier=w44, timeout in ms (-1)=0) -> (notification=w43:bool)  [unwired: 2 in, 3 out]
      }
    }
    n163 = node-c288() -> ()  [unwired: 1 in, 1 out]
  }
  n164 = node-c288(w15) -> ()  [unwired: 1 out]
  n165 = call <vilib>:"Clear Errors.vi"("error in (no error)"=w6) -> ("error out"=w10:errorcluster)  [unwired: 6 in]
  n166 = TCP Close Connection(connection ID=w5, error in (no error)=w10) -> (error out=→"error out":errorcluster)  [unwired: 1 in, 1 out]
